vi "Get Session Error.vi"(8 "error in (no error)":errorcluster, 11 "Sift Stream in":refnum<class "Sift Stream.lvclass">) -> (0 "error out":errorcluster, 1 "Stop Notifier":refnum<notifier>, 2 "session error":errorcluster, 3 "Sift Stream out":refnum<class "Sift Stream.lvclass">)   [LabVIEW 2024, in "Sift Stream.lvlib" / "Sift Stream.lvclass"]
doc: "Gets the stored Session Error and Stop Notifier reference from the plugin."
uses:
  Sift Stream.lvclass
  Sift Stream.lvclass/Sift Stream.ctl
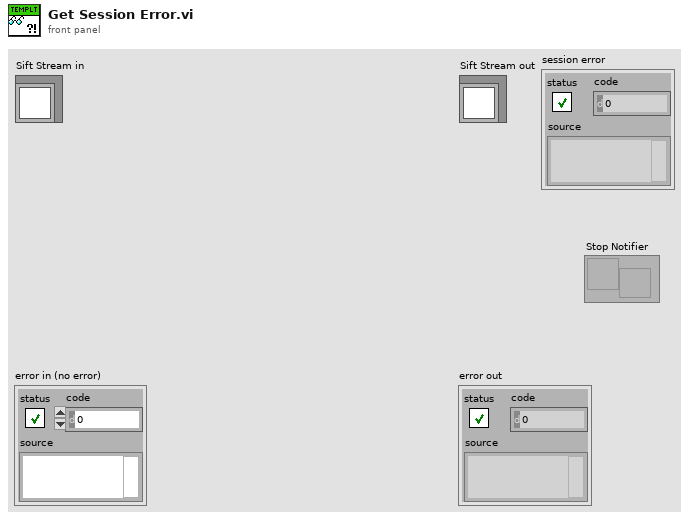
[diagram p1: front panel]
types:
  T1 = typedef "Sift Stream.lvlib/Sift Stream.lvclass/Sift Stream Parameters.ctl" = cluster{"API gRPC URL":string, "API REST URL":string, "API Key":string, "Asset Name":string, "Data Rate":dbl, "Stream Names":string[], "Sift Client":refnum<class "Sift Client.lvclass">, "Session Error":errorcluster, "Stop Notifier":refnum<notifier>, "Channel Name Prefix":string}
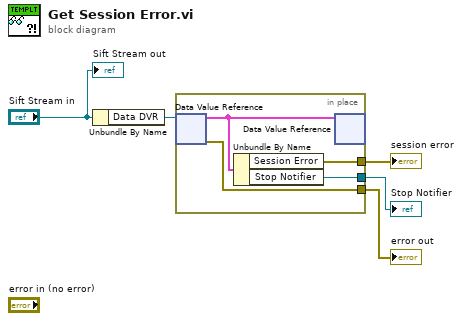
[diagram p0: block diagram]
diagram:
  n1 = Unbundle By Name("Sift Stream in") -> ("Data DVR"=w1:refnum<data-value>)
  n2 = in-place {
    in-place-border: [w9] -> w3
    in-place-border: [w8] -> w5
    in-place-border: [w6] -> w2
    n3 = in-place-dvr #1(w1) -> (w7:T1, w8:errorcluster)
    n4 = Unbundle By Name(w7) -> ("Session Error"=w9:errorcluster, "Stop Notifier"=w6:refnum<notifier>)
    n5 = in-place-dvr #1(w7) -> ()  [unwired: 2 out]
  }
  "error out" <- w5
  "session error" <- w3
  "Stop Notifier" <- w2
  "Sift Stream out" <- "Sift Stream in"
